vi "Set DUT Setup Parameters.vi"(8 "error in (no error)":errorcluster, 11 "Generic DUT Setup in":refnum<class "Generic DUT Setup.lvclass">) -> (0 "error out":errorcluster, 3 "Generic DUT Setup out":refnum<class "Generic DUT Setup.lvclass">)   [LabVIEW 2018, in "Generic DUT Setup.lvlib" / "Generic DUT Setup.lvclass"]
uses:
  Generic DUT Setup.lvclass
  C:/Sequence Automation/Plugins/Measurement Interface.lvlibp/Measurement Interface.lvclass
  Generic DUT Setup.lvclass/Generic DUT Setup.ctl
  Read Sequence Call Step.vi
  Plugins/Measurement Interface.lvlibp/Private Methods/Measurement Parameters/Read Measurement Parameters.vi
  Plugins/String Database.lvlibp/String Database.lvclass
  Plugins/TestStand API Tools (TSAT).lvlibp/Step Actions/TSAT Step Actions.lvlib
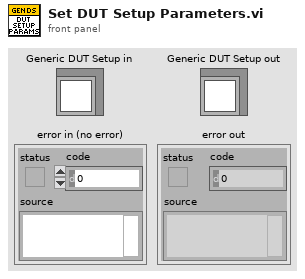
[diagram p1: front panel]
types:
  T1 = typedef "Sequence Call Step Dictionary.lvlibp/Sequence Call Step Dictionary.lvclass/Sequence Call Step.ctl" = cluster{"Sequence Call Step Reference":refnum<k7>, "Sequence Call Parameters":T2[]}
  T2 = typedef "Sequence Call Step Dictionary.lvlibp/Sequence Call Step Dictionary.lvclass/Parameter.ctl" = cluster{"Name":string, "PropertyObject Type":enum16{"Container", "String", "Boolean", "Number", "NamedType", "Reference", "Array", "Aperture Time"}}
  T3 = enum16{"Container", "String", "Boolean", "Number", "NamedType", "Reference", "Array", "Aperture Time"}
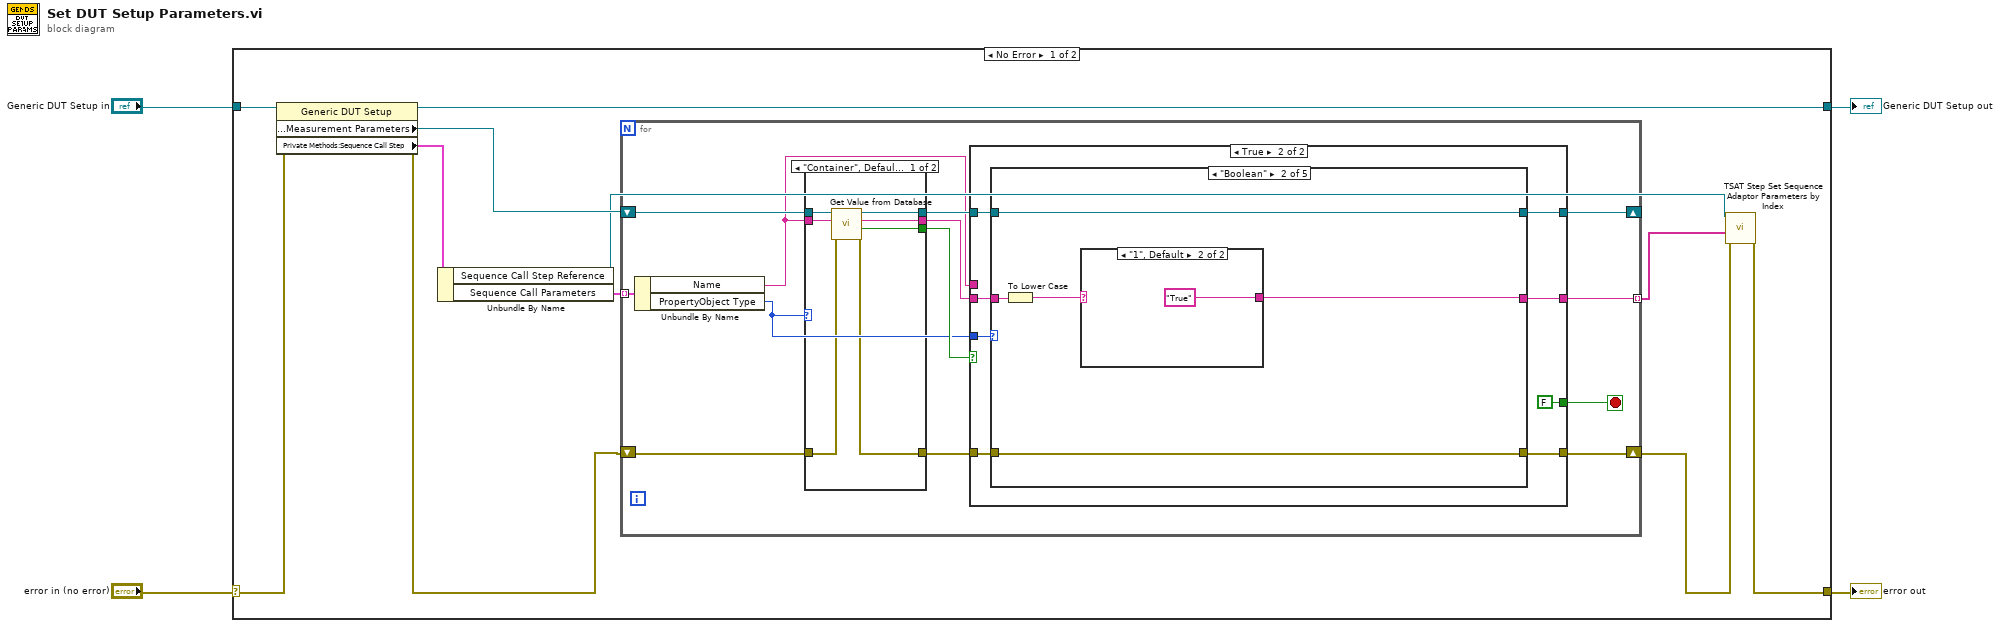
[diagram p0: block diagram]
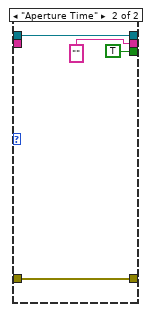
[diagram p2: hidden frame]
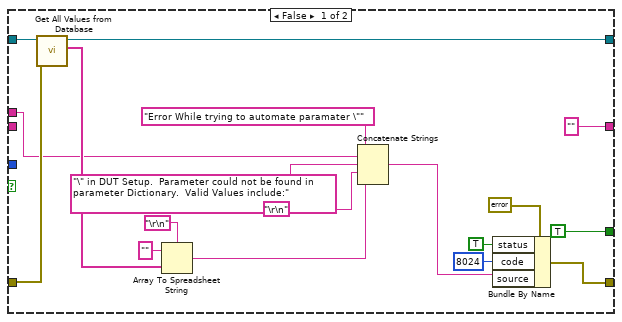
[diagram p3: hidden frame]
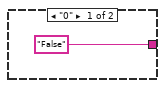
[diagram p5: hidden frame]
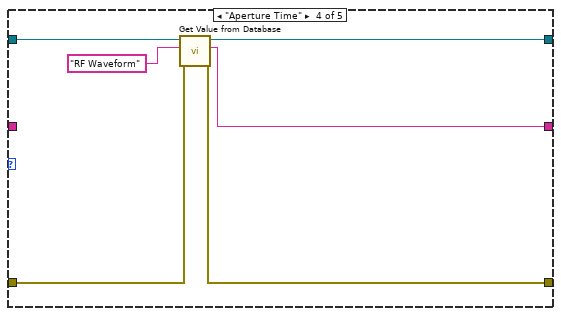
[diagram p7: hidden frame]
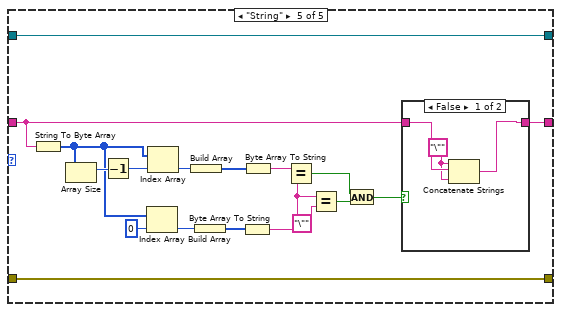
[diagram p8: hidden frame]
diagram:
  n1 = case shown="No Error" "error in (no error)" {
    selector: "error in (no error)" -> [w15 w108]
    tunnel: [w9 w108] -> w3
    tunnel: [w13 w107] -> w1
    tunnel: "Generic DUT Setup in" -> [w14 w107]
    frame No Error {
      n2 = property class="Generic DUT Setup"(reference=w14, error in=w15) -> (reference out=w13:refnum<class "Generic DUT Setup.lvclass">, error out=w6:errorcluster, "Protected Methods:Measurement Parameters"=w11:refnum<class "String Database.lvclass">, "Private Methods:Sequence Call Step"=w12:T1)
      n3 = Unbundle By Name(w12) -> ("Sequence Call Step Reference"=w8:refnum<k7>, "Sequence Call Parameters"=w10:T2[])
      n4 = for {
        tunnel: w10 -> [w28] mode=indexing
        shift-right: [w22] -> w5
        shift-left: w6 -> [w27]
        shift-right: [w20] -> _
        shift-left: w11 -> [w26]
        tunnel: [w23] -> w7 mode=indexing
        stop <- w18 stop-if-true
        n5 = Unbundle By Name(w28) -> ("Name"=w17:string, "PropertyObject Type"=w16:T3)
        n6 = case shown="\"Container\", Default" w16 {
          tunnel: w27 -> [w35 w38]
          tunnel: w26 -> [w34 w39]
          tunnel: [w33 "" ("Entry Value")] -> w25
          tunnel: [w32 TRUE ("Entry Found")] -> w24
          tunnel: [w31 w38] -> w21
          tunnel: [w30 w39] -> w19
          tunnel: w17 -> [w29 _]
          frame "Container", Default {
            n7 = call "Get Value from Database.vi"("error in (no error)"=w35, "Entry Name"=w29, "Message in"=w34) -> ("error out"=w31:errorcluster, "Entry Found"=w32:bool, "Entry Value"=w33:string, "Message out"=w30:refnum<class "String Database.lvclass">)  [unwired: 5 in]
          }
          frame "Aperture Time" {
          }
        }
        n8 = case shown="True" w24 {
          tunnel: w25 -> [_ w65]
          tunnel: ["" ("Entry Value") w64] -> w23
          tunnel: [w57 w61] -> w22
          tunnel: w21 -> [w47 w62]
          tunnel: [w48 w60] -> w20
          tunnel: w19 -> [w49 w59]
          tunnel: [TRUE ("status") FALSE ("status")] -> w18
          tunnel: w17 -> [w40 _]
          tunnel: w16 -> [_ w58]
          frame False {
            n9 = call "Get All Values from Database.vi"("error in (no error)"=w47, "String Database in"=w49) -> ("Names"=w41:string[], "String Database out"=w48:refnum<class "String Database.lvclass">)  [unwired: 6 in, 2 out]
            n10 = Array To Spreadsheet String(delimiter (Tab)="\r\n", array=w41, 3:"" ("format string")) -> (spreadsheet string=w44:string)
            n11 = Concatenate Strings("Error While trying to automate paramater \"", w40, "\" in DUT Setup.  Parameter could not be found in parameter Dictionary.  Valid Values include:" ("string"), "\r\n", w44) -> (w51:string)
            n12 = Bundle By Name(cluster=errorcluster {"status"=FALSE, "code"=0, "source"=""} ("error out"), "status"=TRUE, "code"=8024, "source"=w51) -> (w57:errorcluster)
          }
          frame True {
            n13 = case shown="\"Boolean\"" w58 {
              tunnel: w65 -> [w68 w71 w78 _ w87]
              tunnel: [w68 w69 w78 w79 w88] -> w64
              tunnel: w62 -> [w67 w73 w77 w83 w86]
              tunnel: [w67 w73 w77 w82 w86] -> w61
              tunnel: [w66 w72 w76 w81 w85] -> w60
              tunnel: w59 -> [w66 w72 w76 w84 w85]
              frame "Container", Default {
              }
              frame "Boolean" {
                n14 = To Lower Case(string=w71) -> (all lower case string=w70:string)
                n15 = case shown="\"1\", Default" w70 {
                  tunnel: ["False" "True"] -> w69
                  frame "0" {
                  }
                  frame "1", Default {
                  }
                }
              }
              frame "Number" {
              }
              frame "Aperture Time" {
                n16 = call "Get Value from Database.vi"("error in (no error)"=w83, "Entry Name"="RF Waveform", "Message in"=w84) -> ("error out"=w82:errorcluster, "Entry Value"=w79:string, "Message out"=w81:refnum<class "String Database.lvclass">)  [unwired: 5 in, 1 out]
              }
              frame "String" {
                n17 = String To Byte Array(string=w87) -> (unsigned byte array=w100:u8[])
                n18 = Array Size(array=w100) -> (size(s)=w102:i32)
                n19 = Decrement(x=w102) -> (x-1=w101:i32)
                n20 = Index Array(array=w100, index=0) -> (element=w98:u8)
                n21 = Index Array(array=w100, index=w101) -> (element=w99:u8)
                n22 = Build Array(w99) -> (w96:u8[])
                n23 = Build Array(w98) -> (w97:u8[])
                n24 = Byte Array To String(unsigned byte array=w97) -> (string=w94:string)
                n25 = Byte Array To String(unsigned byte array=w96) -> (string=w95:string)
                n26 = Equal?(x=w95, y=w94) -> (x = y?=w91:bool)
                n27 = Equal?(x=w94, y="\"") -> (x = y?=w92:bool)
                n28 = And(x=w91, y=w92) -> (x .and. y?=w89:bool)
                n29 = case shown="False" w89 {
                  tunnel: [w104 w106] -> w88
                  tunnel: w87 -> [w105 w106]
                  frame False {
                    w103 = "\"" ("string")
                    n30 = Concatenate Strings(w103, w105, w103) -> (w104:string)
                  }
                  frame True {
                  }
                }
              }
            }
          }
        }
      }
      n31 = call "TSAT Step Set Sequence Adaptor Parameters by Index.vi"("error in"=w5, "Parameter Array"=w7, "Step In"=w8) -> ("Error Out"=w9:errorcluster)  [unwired: 7 in, 1 out]
    }
    frame Error {
    }
  }
  "error out" <- w3
  "Generic DUT Setup out" <- w1
